vi "Actor Core.vi"(8 "error in":errorcluster, 11 "Fancy Entry Console View In":refnum<class "Extra Fancy Entry Console View.lvclass">) -> (0 "error out":errorcluster, 3 "Actor out":refnum<class "Actor.lvclass">)   [LabVIEW 2019, in "Extra Fancy Entry Console View.lvclass"]
doc: "(<B>Filename</B>: Actor Framework.lvlib:Actor.lvclass:Actor Core.vi)\n\nReceives messages to the actor, reacts to them, and initiates any error handling that may shut the actor down.\n\nDescendant classes may override this VI to append parallel tasks for the actor to complete while it handles messages. Overrides use the Call Parent Method node.\n\n<License>\nCopyright © 2017 Composed Systems, LLC | All rights reserved\nwww.composed.io\n\nAuthor: Ethan Stern <ethan.stern@composed.io>\n\nThis software is provided \"AS IS\" WITHOUT WARRANTIES, either express or implied, AND IS FOR EDUCATIONAL PURPOSES ONLY.\n</License>"
uses:
  <vilib>/gpm_packages/@cs/Car-wash/Source/Extra Fancy Entry Console View/Extra Fancy Entry Console View.lvclass
  C:/Program Files/National Instruments/LabVIEW 2019/vi.lib/gpm_packages/@cs/Car-wash/Source/Entry Console View Definition/Entry Console View Definition/Entry Console View Definition.lvclass
  <vilib>/ActorFramework/Actor/Actor.lvclass
  <vilib>/gpm_packages/@cs/Car-wash/Source/Entry Console View Definition/Entry Console View Definition/Entry Console View Definition.lvclass
panel:
  in  "Start Macro":bool
  in  "20 Dollar Option":bool
  in  "10 Dollar Option":bool
  in  "5 Dollar Option":bool
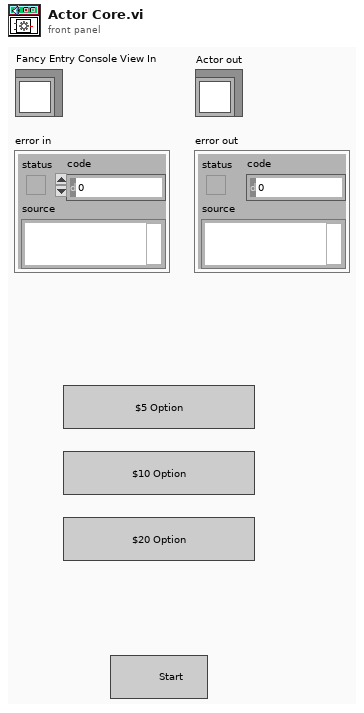
[diagram p1: front panel]
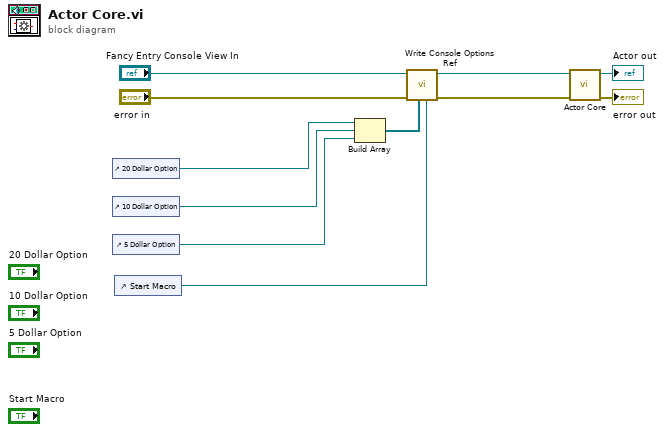
[diagram p0: block diagram]
diagram:
  n1 = control-ref of="20 Dollar Option"() -> (w5:refnum<vi>)
  n2 = control-ref of="10 Dollar Option"() -> (w4:refnum<vi>)
  n3 = control-ref of="5 Dollar Option"() -> (w2:refnum<vi>)
  n4 = control-ref of="Start Macro"() -> (w1:refnum<vi>)
  n5 = Build Array(w5, w4, w2) -> (w3:refnum<vi>[])
  n6 = call <vilib>:"Write Console Options Ref.vi"("Start Ref"=w1, "Console Options"=w3, "Entry Console View Definition in"="Fancy Entry Console View In") -> ("Entry Console View Definition out"=w6:refnum<class "Extra Fancy Entry Console View.lvclass">)  [unwired: 8 in]
  n7 = call-parent "Actor Core.vi"("error in"="error in", "Entry Console View Definition In"=w6) -> ("error out"=→"error out":errorcluster, "Actor out"=→"Actor out":refnum<class "Actor.lvclass">)  [unwired: 8 in]
